vi "转速_反馈.vi"(10 "最高转速":i32, 11 "unsigned byte array":u8[](array[numeric])) -> (2 "转速反馈":dbl format="%#_4g")   [LabVIEW 2012]
panel:
  out "x+y 2":i32
  out "布尔数组":bool[](array[boolean])
  out "x+y":u16 format="%b"
  out "x*y":dbl
  out "元素 2":u8
  out "元素":u16
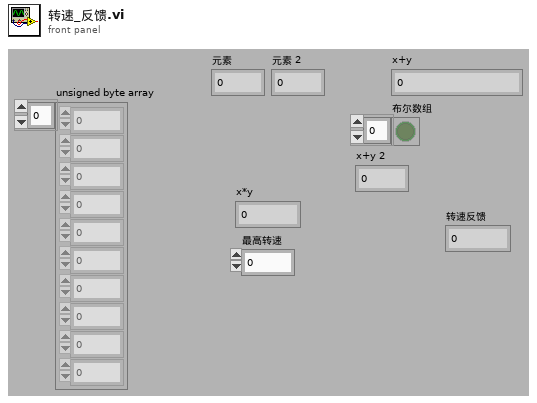
[diagram p1: front panel]
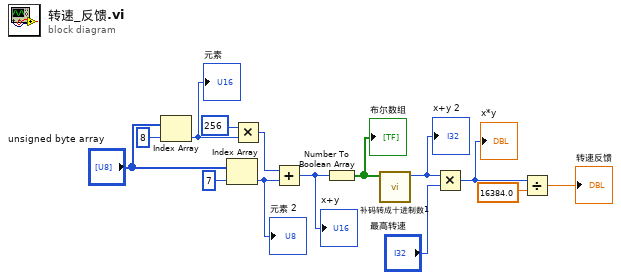
[diagram p0: block diagram]
diagram:
  n1 = Index Array(array="unsigned byte array", index=8 ("索引")) -> (element=w9:u8)
  "元素" <- w9
  n2 = Index Array(array="unsigned byte array", index=7 ("索引")) -> (element=w12:u8)
  "元素 2" <- w12
  n3 = Multiply(x=u16 256, y=w9) -> (x*y=w11:u16)
  n4 = Add(x=w11, y=w12) -> (x+y=w4:u16)
  "x+y" <- w4
  n5 = Number To Boolean Array(number=w4) -> (Boolean array=w1:bool[])
  "布尔数组" <- w1
  n6 = call "补码转成十进制数1.vi"("数组"=w1) -> ("x+y 2"=w2:i16)  [unwired: 10 in]
  "x+y 2" <- w2
  n7 = Multiply(x=w2, y="最高转速") -> (x*y=w13:i32)
  "x*y" <- w13
  n8 = Divide(x=w13, y=16384.0) -> (x/y=→"转速反馈":dbl)
